vi "Terminal_Random_Select.vi"(10 "数组":dbl[][](array[numeric])) -> (2 "添加的数组":dbl[](array[numeric]))   [LabVIEW 2014]
panel:
  out "元素 3":dbl
  out "元素 2":i32
  out "元素":i32
  out "数组 2":dbl[][](array[numeric])
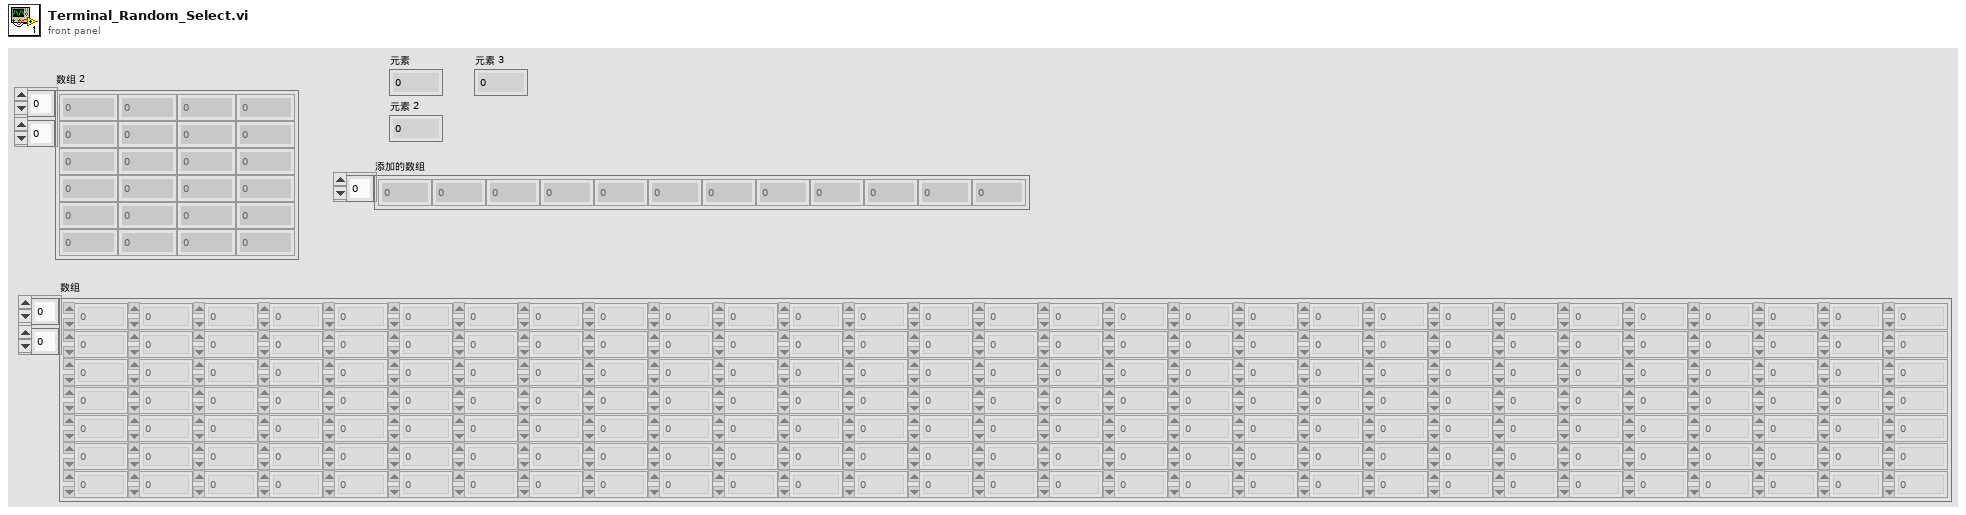
[diagram p1: front panel]
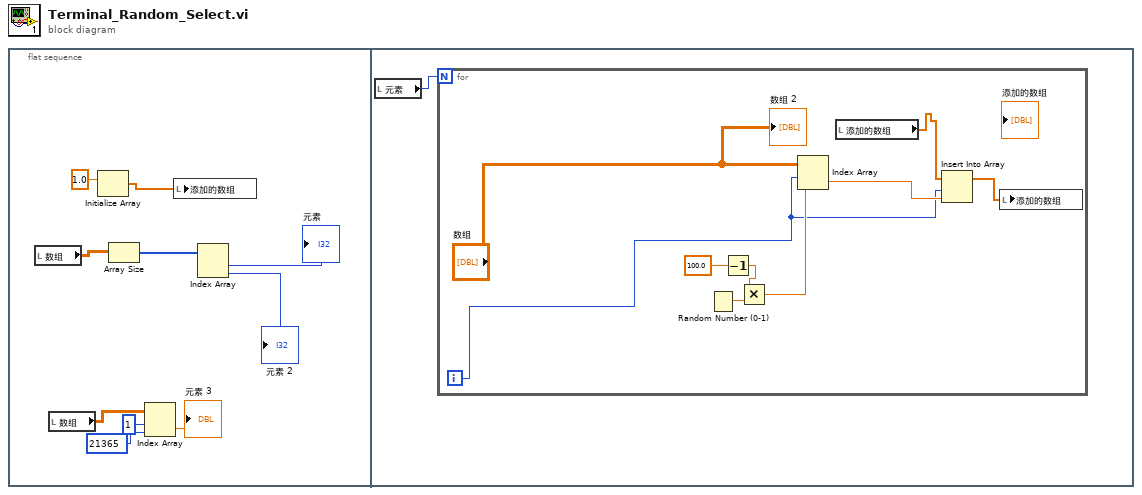
[diagram p0: block diagram]
diagram:
  n1 = flat-sequence {
    frame #0 {
      n2 = local read "数组"() -> (w8:dbl[][])
      n3 = local read "数组"() -> (w4:dbl[][])
      n4 = Initialize Array(1.0 ("元素")) -> (w10:dbl[])  [unwired: 1 in]
      n5 = Array Size(array=w8) -> (size(s)=w7:i32[])
      n6 = Index Array(array=w4, index (row)=1 ("索引 (行)"), index (col)=21365 ("禁用的索引 (列)")) -> (element=→"元素 3":dbl)
      n7 = local write "添加的数组"(w10) -> ()
      n8 = Index Array(array=w7) -> (element #1=→"元素":i32, element #2=→"元素 2":i32)  [unwired: 2 in]
    }
    frame #1 {
      n9 = local read "元素"() -> (w11:i32)
      n10 = for {
        N: w11 -> [_]
        i -> [w13]
        n11 = Random Number (0-1)() -> (number: 0 to 1=w17:dbl)
        n12 = Decrement(x=100.0) -> (x-1=w14:dbl)
        n13 = Multiply(x=w14, y=w17) -> (x*y=w15:dbl)
        n14 = Index Array(array="数组", index (row)=w13, index (col)=w15) -> (element=w19:dbl)
        n15 = local read "添加的数组"() -> (w16:dbl[])
        n16 = Insert Into Array(array=w16, index=w13, new element=w19) -> (w18:dbl[])
        n17 = local write "添加的数组"(w18) -> ()
        "数组 2" <- "数组"
      }
    }
  }
